vi "get value for key.vi"(8 "error in":errorcluster, 10 "key":string, 11 "fixed channel configuration in":refnum<class "ScaleAndLimitModule configuration.lvclass">) -> (0 "error out":errorcluster, 1 "value":string, 3 "fixed channel configuration out":refnum<class "ScaleAndLimitModule configuration.lvclass">)   [LabVIEW 2017, in "ScaleAndLimitModule configuration.lvclass"]
uses:
  ScaleAndLimitModule configuration.lvclass
  <vilib>/NI/DCAF/Tag Editor Core/control module/configuration/control module configuration.lvclass
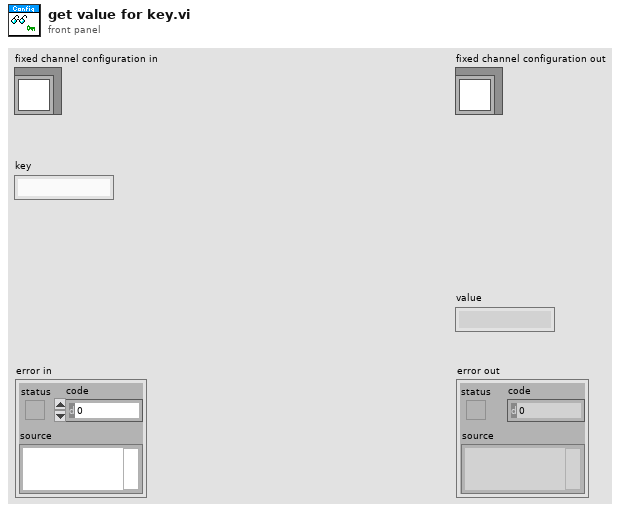
[diagram p1: front panel]
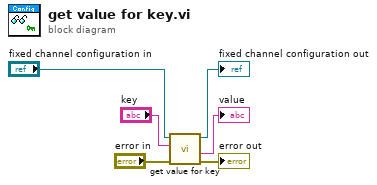
[diagram p0: block diagram]
diagram:
  n1 = call-parent "get value for key.vi"("error in"="error in", "key"="key", "fixed channel configuration in"="fixed channel configuration in") -> ("error out"=→"error out":errorcluster, "value"=→"value":string, "fixed channel configuration out"=→"fixed channel configuration out":refnum<class "ScaleAndLimitModule configuration.lvclass">)  [unwired: 6 in]
